vi "Run Test.vi"(8 "error in (no error)":errorcluster, 11 "Thermal Test in":refnum<class "Thermal Test.lvclass">) -> (0 "error out":errorcluster, 3 "Thermal Test out":refnum<class "Thermal Test.lvclass">)   [LabVIEW 2023, in "Thermal Test.lvclass"]
uses:
  Thermal Test.lvclass
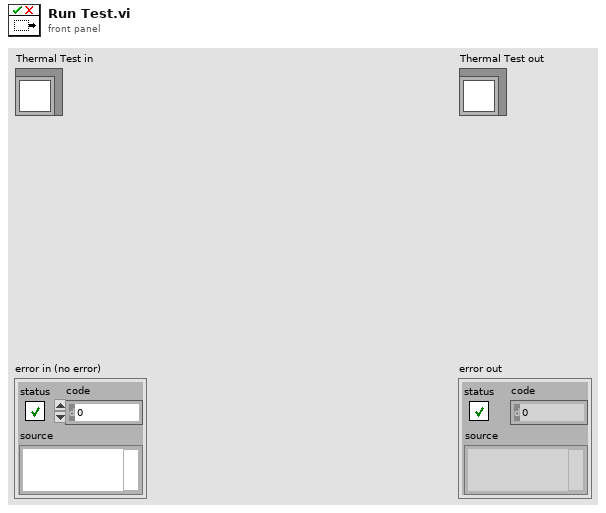
[diagram p1: front panel]
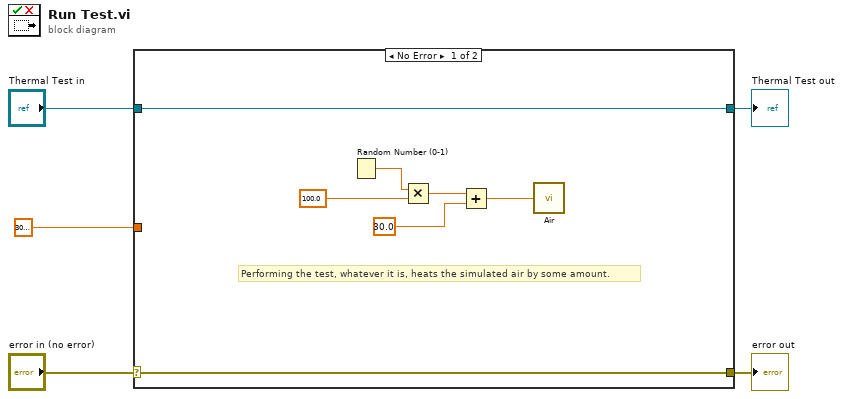
[diagram p0: block diagram]
diagram:
  n1 = case shown="No Error" "error in (no error)" {
    selector: "error in (no error)" -> [w11 w14]
    tunnel: [w11 w14] -> w4
    tunnel: [w12 w13] -> w2
    tunnel: "Thermal Test in" -> [w12 w13]
    tunnel: dbl[unit] 303.15 ("y") -> [_ _]
    frame No Error {
      # "Performing the test, whatever it is, heats the simulated air by some amount."
      n2 = Random Number (0-1)() -> (number: 0 to 1=w10:dbl)
      n3 = Multiply(x=w10, y=dbl[unit] 100.0) -> (x*y=w9:dbl[unit])
      n4 = Add(x=w9, y=dbl[unit] 30.0) -> (x+y=w8:dbl[unit])
      n5 = call "Air.vi"("temperature adjustment"=w8) -> ()  [unwired: 1 out]
    }
    frame Error {
    }
  }
  "error out" <- w4
  "Thermal Test out" <- w2
